vi "Serialize.vi"(8 "error in":errorcluster, 9 "OwningElement in":refnum<k20>, 10 "Document in":refnum<k20>, 11 "OperationCycle in":refnum<class "OperationCycle.lvclass">) -> (0 "error out":errorcluster, 1 "OwningElement out":refnum<k20>, 2 "Document out":refnum<k20>, 3 "OperationCycle out":refnum<class "OperationCycle.lvclass">)   [LabVIEW 2021, in "ProligentXMLGenerator.lvlib" / "OperationCycle.lvclass"]
uses:
  OperationCycle.lvclass
  OperationCycle.lvclass/OperationCycle.ctl
  <vilib>/xml/NI_XML.lvlib
  Base/DOMSupport/DOMSupport.lvlib
  Model/CustomData/CustomData.lvclass
  <vilib>/xml/Close Reference(Node).vi
  Base/ProcessFullName/ProcessFullName.lvclass
  C:/Projects/proligent-xml-generator-labview/src/ProligentXMLGenerator/Base/NonEmptyString/NonEmptyString.lvclass
  C:/Projects/proligent-xml-generator-labview/src/ProligentXMLGenerator/Base/String/String.lvclass
  C:/Projects/proligent-xml-generator-labview/src/ProligentXMLGenerator/Base/Attribute/Attribute.lvclass
  C:/Projects/proligent-xml-generator-labview/src/ProligentXMLGenerator/Base/ProcessFullName/ProcessFullName.lvclass
  Base/NonEmptyString_64/NonEmptyString_64.lvclass
  C:/Projects/proligent-xml-generator-labview/src/ProligentXMLGenerator/Base/NonEmptyString_64/NonEmptyString_64.lvclass
  Base/Guid/Guid.lvclass
  C:/Projects/proligent-xml-generator-labview/src/ProligentXMLGenerator/Base/Guid/Guid.lvclass
  Base/NonEmptyString_65/NonEmptyString_65.lvclass
  C:/Projects/proligent-xml-generator-labview/src/ProligentXMLGenerator/Base/NonEmptyString_65/NonEmptyString_65.lvclass
  Base/FullName/FullName.lvclass
  C:/Projects/proligent-xml-generator-labview/src/ProligentXMLGenerator/Base/FullName/FullName.lvclass
  Base/NonEmptyString_255/NonEmptyString_255.lvclass
  C:/Projects/proligent-xml-generator-labview/src/ProligentXMLGenerator/Base/NonEmptyString_255/NonEmptyString_255.lvclass
  Base/ExecutionStatus/ExecutionStatus.lvclass
  C:/Projects/proligent-xml-generator-labview/src/ProligentXMLGenerator/Base/ExecutionStatus/ExecutionStatus.lvclass
  Base/DateTime/DateTime.lvclass
  C:/Projects/proligent-xml-generator-labview/src/ProligentXMLGenerator/Base/DateTime/DateTime.lvclass
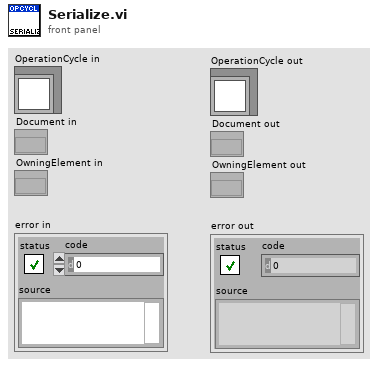
[diagram p1: front panel]
types:
  T1 = typedef "ProligentXMLGenerator.lvlib/OperationCycle.lvclass/Data.ctl" = cluster{"Name":string, "CustomData":refnum<class "CustomData.lvclass">, "ProcessFullName":refnum<class "ProcessFullName.lvclass">, "ProcessVersion":refnum<class "NonEmptyString_64.lvclass">, "OperationCycleId":refnum<class "Guid.lvclass">, "OperationName":refnum<class "NonEmptyString_65.lvclass">, "Location":refnum<class "FullName.lvclass">, "User":refnum<class "NonEmptyString_255.lvclass">, "OperationCycleStatus":refnum<class "ExecutionStatus.lvclass">, "OperationCycleStartTime":refnum<class "DateTime.lvclass">, "OperationCycleEndTime":refnum<class "DateTime.lvclass">, "TimeZoneInfoId":string}
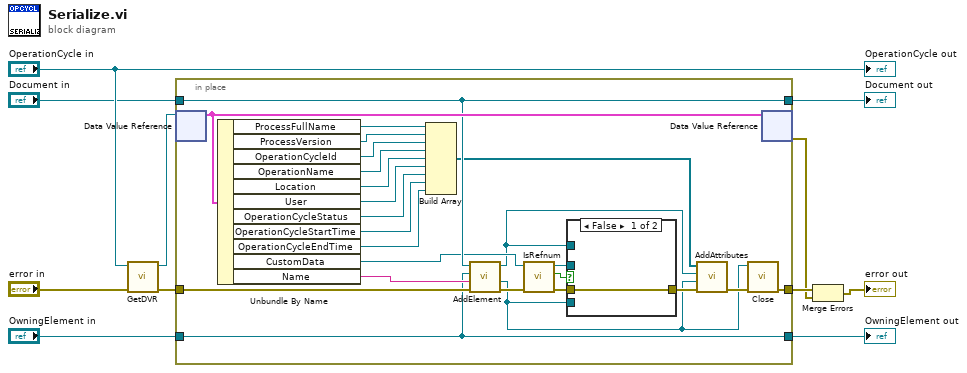
[diagram p0: block diagram]
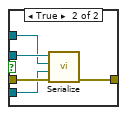
[diagram p2: hidden frame]
diagram:
  n1 = call "GetDVR.vi"("error in"="error in", "OperationCycle in"="OperationCycle in") -> ("error out"=w3:errorcluster, "DVRReference"=w2:refnum<data-value>)  [unwired: 8 in]
  n2 = in-place "In Place Element Structure" {
    in-place-border: [w36] -> w4
    in-place-border: "Document in" -> [w31]
    in-place-border: w3 -> [w35]
    in-place-border: "OwningElement in" -> [w33]
    in-place-border: [w33] -> w6
    in-place-border: [w31] -> w5
    n3 = in-place-dvr #1(w2) -> (w32:T1)  [unwired: 1 out]
    n4 = Unbundle By Name(w32) -> ("ProcessFullName"=w30:refnum<class "ProcessFullName.lvclass">, "ProcessVersion"=w22:refnum<class "NonEmptyString_64.lvclass">, "OperationCycleId"=w21:refnum<class "Guid.lvclass">, "OperationName"=w29:refnum<class "NonEmptyString_65.lvclass">, "Location"=w20:refnum<class "FullName.lvclass">, "User"=w28:refnum<class "NonEmptyString_255.lvclass">, "OperationCycleStatus"=w27:refnum<class "ExecutionStatus.lvclass">, "OperationCycleStartTime"=w26:refnum<class "DateTime.lvclass">, "OperationCycleEndTime"=w23:refnum<class "DateTime.lvclass">, "CustomData"=w19:refnum<class "CustomData.lvclass">, "Name"=w34:string)
    n5 = Build Array(w30, w22, w21, w29, w20, w28, w27, w26, w23) -> (w25:refnum<class "Attribute.lvclass">[])
    n6 = call "AddElement.vi"("error in"=w35, "Name"=w34, "OwningElement in"=w33, "Document in"=w31) -> ("error out"=w18:errorcluster, "NewElement"=w13:refnum<k20>, "Document out"=w12:refnum<k20>)  [unwired: 4 in, 1 out]
    n7 = call "IsRefnum.vi"("error in"=w18, "CustomDataType in"=w19) -> ("error out"=w16:errorcluster, "IsRefnum"=w17:bool, "CustomDataType out"=w14:refnum<class "CustomData.lvclass">)  [unwired: 7 in]
    n8 = case shown="False" w17 {
      tunnel: w16 -> [w37 w42]
      tunnel: [w37 w41] -> w15
      tunnel: w14 -> [_ w40]
      tunnel: w13 -> [_ w39]
      tunnel: w12 -> [_ w38]
      frame False {
      }
      frame True {
        n9 = call "Serialize.vi"("error in"=w42, "OwningElement in"=w39, "Document in"=w38, "CustomDataType in"=w40) -> ("error out"=w41:errorcluster)  [unwired: 4 in, 3 out]
      }
    }
    n10 = call "AddAttributes.vi"("error in"=w15, "OwningElement in"=w13, "Document in"=w12, "Attributes"=w25) -> ("error out"=w24:errorcluster)  [unwired: 5 in, 2 out]
    n11 = call-poly <vilib>:"Close.vi"("error in (no error)"=w24, "node"=w13) -> ("error out"=w36:errorcluster)  [unwired: 7 in]
    n12 = in-place-dvr #1(w32) -> (w1:errorcluster)  [unwired: 1 out]
  }
  "Document out" <- w5
  "OwningElement out" <- w6
  n13 = Merge Errors(w4, w1) -> (→"error out":errorcluster)
  "OperationCycle out" <- "OperationCycle in"
